vi "Set Shared Library Name.vi"(8 "error in (no error)":errorcluster, 10 "Shared library file name":string, 11 "DLL in":refnum<class "NI_AB_API_DLL.lvclass">) -> (0 "error out":errorcluster, 3 "DLL out":refnum<class "NI_AB_API_DLL.lvclass">)   [LabVIEW 2020, in "NI_AB_API_DLL.lvclass"]
uses:
  <vilib>/AppBuilder/AB_API/DLL/NI_AB_API_DLL.lvclass
  e:/builds/penguin/labview/branches/2020/dev/dist/vi.lib/AppBuilder/AB_API/Build/NI_AB_API_Build.lvclass
  <vilib>/AppBuilder/AB_Classes/DLL/AB_DLL.lvclass
  e:/builds/penguin/labview/branches/2020/dev/dist/vi.lib/AppBuilder/AB_Classes/TargetFile/AB_Targetfile.lvclass
  e:/builds/penguin/labview/branches/2020/dev/dist/vi.lib/AppBuilder/AB_Classes/Build/AB_Build.lvclass
  <resource>/Framework/Providers/Common/provcom_StringGlobals.vi
  <vilib>/AppBuilder/AB_API/Build/NI_AB_API_Build.lvclass
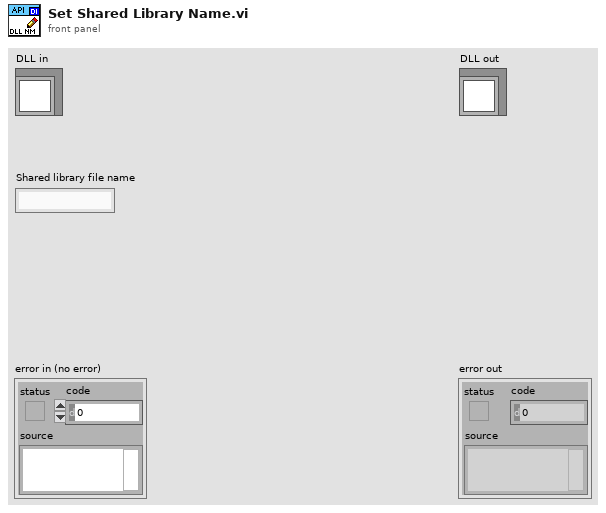
[diagram p1: front panel]
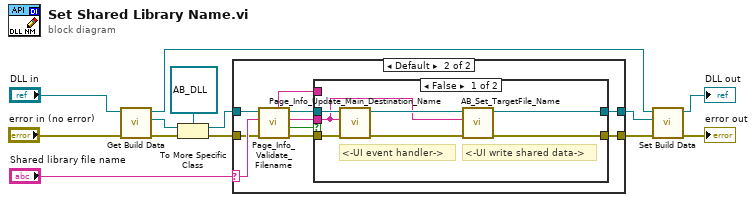
[diagram p0: block diagram]
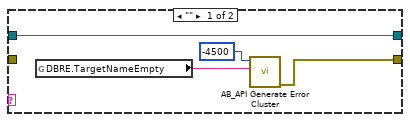
[diagram p2: hidden frame]
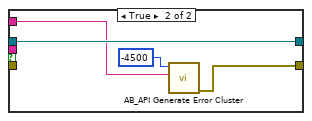
[diagram p3: hidden frame]
diagram:
  n1 = call <vilib>:"Get Build Data.vi"("error in (no error)"="error in (no error)", "NI_AB_API_Build in"="DLL in") -> ("error out"=w5:errorcluster, "AB_Build.lvclass"=w3:refnum<class "AB_Build.lvclass">, "NI_AB_API_Build out"=w8:refnum<class "NI_AB_API_DLL.lvclass">)  [unwired: 7 in]
  n2 = To More Specific Class(target class=refnum<class "AB_DLL.lvclass"> refnum ("AB_DLL.lvclass"), reference=w3, error in=w5) -> (specific class reference=w2:refnum<class "AB_DLL.lvclass">, error out=w4:errorcluster)
  n3 = case shown="Default" "Shared library file name" {
    selector: "Shared library file name" -> [_ w23]
    tunnel: [w15 w27] -> w7
    tunnel: w4 -> [_ w20]
    tunnel: w2 -> [w14 w25]
    tunnel: [w14 w26] -> w6
    frame "" {
      n4 = global read "provcom_StringGlobals.vi" "DBRE.TargetNameEmpty"() -> (w16:string)
      n5 = call <vilib>:"AB_API Generate Error Cluster.vi"("Additional Message"=w16, "Code"=-4500) -> ("error out"=w15:errorcluster)  [unwired: 9 in]
    }
    frame Default {
      n6 = call-dynamic "Page_Info_Validate_Filename.vi"("error in (no error)"=w20, "Filename in"=w23, "AB_DLL in"=w25) -> ("error out"=w19:errorcluster, "hasInvalidCharacters"=w21:bool, "Filename out"=w22:string, "AB_DLL out"=w24:refnum<class "AB_DLL.lvclass">, "message"=w18:string)  [unwired: 4 in]
      n7 = case shown="False" w21 {
        tunnel: [w33 w37] -> w27
        tunnel: w19 -> [w31 _]
        tunnel: w24 -> [w30 w36]
        tunnel: [w34 w36] -> w26
        tunnel: w22 -> [w28 _]
        tunnel: w18 -> [_ w35]
        frame False {
          # "<-UI write shared data->"
          # "<-UI event handler->"
          n8 = call-dynamic "Page_Info_Update_Main_Destination_Name.vi"("error in (no error)"=w31, "destination name"=w28, "AB_Build in"=w30) -> ("error out"=w32:errorcluster, "AB_Build out"=w29:refnum<class "AB_DLL.lvclass">)  [unwired: 7 in]
          n9 = call <vilib>:"AB_Set_TargetFile_Name.vi"("error in (no error)"=w32, "Target filename"=w28, "TargetFile in"=w29) -> ("error out"=w33:errorcluster, "TargetFile out"=w34:refnum<class "AB_DLL.lvclass">)  [unwired: 7 in]
        }
        frame True {
          n10 = call <vilib>:"AB_API Generate Error Cluster.vi"("Additional Message"=w35, "Code"=-4500) -> ("error out"=w37:errorcluster)  [unwired: 9 in]
        }
      }
    }
  }
  n11 = call <vilib>:"Set Build Data.vi"("error in (no error)"=w7, "AB_Build.lvclass"=w6, "NI_AB_API_Build in"=w8) -> ("error out"=→"error out":errorcluster, "NI_AB_API_Build out"=→"DLL out":refnum<class "NI_AB_API_DLL.lvclass">)  [unwired: 7 in]
